vi "Module Cleanup.vi"(8 "error in (no error)":errorcluster, 11 "Hardware Info Module in":refnum<class "Hardware Info Module.lvclass">) -> (0 "error out":errorcluster, 3 "Hardware Info Module out":refnum<class "Hardware Info Module.lvclass">)   [LabVIEW 2020, in "Volatus.lvlib" / "Hardware Info Module.lvclass"]
uses:
  Hardware Info Module.lvclass
  Hardware Info Module.lvclass/Hardware Info Module.ctl
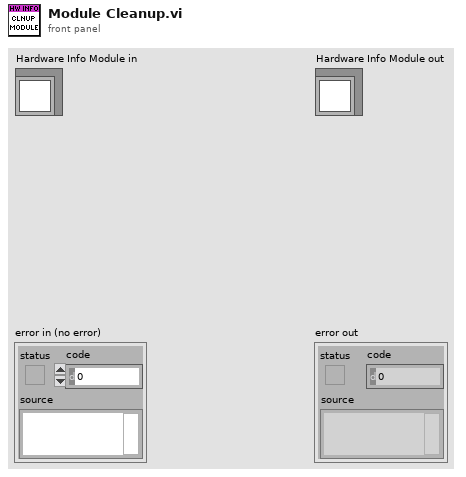
[diagram p1: front panel]
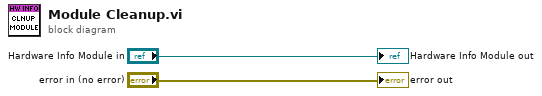
[diagram p0: block diagram]
diagram:
  "error out" <- "error in (no error)"
  "Hardware Info Module out" <- "Hardware Info Module in"
